vi "Backup File.vi"(7 "Delete Origin File?":bool=TRUE, 8 "error in":errorcluster, 10 "Backup Directory":path, 11 "Original File Path in":path) -> (0 "error out":errorcluster, 3 "Backup File Path out":path)   [LabVIEW 2021, in "EDT File IO.lvlib"]
uses:
  EDT File IO.lvlib
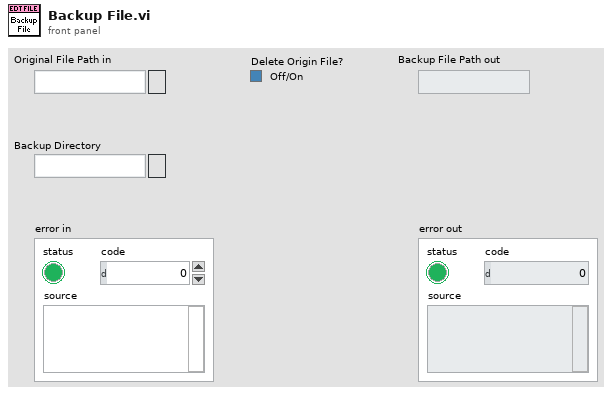
[diagram p1: front panel]
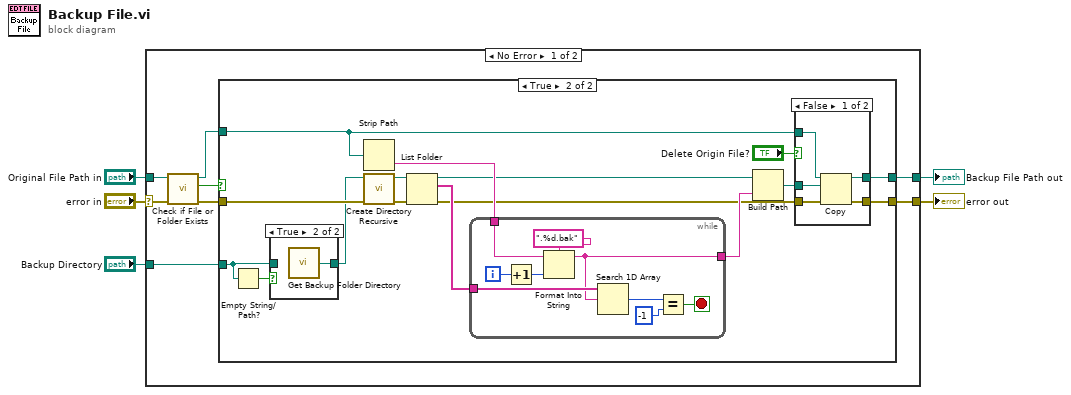
[diagram p0: block diagram]
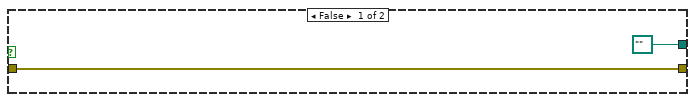
[diagram p2: hidden frame]
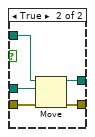
[diagram p3: hidden frame]
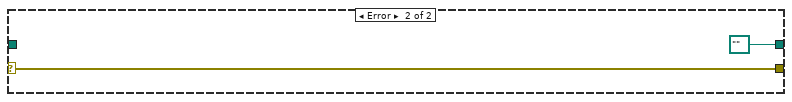
[diagram p5: hidden frame]
diagram:
  n1 = case shown="No Error" "error in" {
    selector: "error in" -> [w9 w54]
    tunnel: [w13 w54] -> w4
    tunnel: [w12 path "" ("File Path in")] -> w3
    tunnel: "Original File Path in" -> [w10 _]
    tunnel: "Backup Directory" -> [w11 _]
    frame No Error {
      n2 = call <vilib>:"Check if File or Folder Exists.vi"("error in (no error)"=w9, "path"=w10) -> ("error out"=w7:errorcluster, "file or folder exists?"=w8:bool, "dup path"=w6:path)  [unwired: 7 in]
      n3 = case shown="True" w8 {
        tunnel: [w15 w31] -> w13
        tunnel: [path "" ("new path") w30] -> w12
        tunnel: w11 -> [_ w24]
        tunnel: w6 -> [_ w23]
        tunnel: w7 -> [w15 w20]
        frame False {
        }
        frame True {
          n4 = Empty String/Path?(string/path=w24) -> (empty?=w25:bool)
          n5 = case shown="True" w25 {
            tunnel: [w42 w43] -> w19
            tunnel: w24 -> [w42 _]
            frame False {
            }
            frame True {
              n6 = call "Get Backup Folder Directory.vi"() -> ("Backup Folder Directory"=w43:path)
            }
          }
          n7 = Strip Path(path=w23) -> (name=w28:string)  [unwired: 1 out]
          n8 = call <vilib>:"Create Directory Recursive.vi"("error in (no error)"=w20, "directory"=w19) -> ("error out"=w17:errorcluster, "directory copy"=w18:path)  [unwired: 3 in, 1 out]
          n9 = List Folder(path=w18, error in=w17) -> (path out=w16:path, filenames=w29:string[], error out=w21:errorcluster)  [unwired: 2 in, 1 out]
          n10 = while {
            tunnel: w29 -> [w52]
            tunnel: w28 -> [w46]
            tunnel: [w44] -> w27
            i -> [w48]
            stop <- w49 stop-if-true
            n11 = Increment(x=w48) -> (x+1=w47:i32)
            n12 = Format Into String(format string=".%d.bak", initial string=w46, w47) -> (resulting string=w44:string)  [unwired: 1 in, 1 out]
            n13 = Search 1D Array(1D array=w52, element=w44) -> (index of element=w51:i32)  [unwired: 1 in]
            n14 = Equal?(x=w51, y=-1) -> (x = y?=w49:bool)
          }
          n15 = Build Path(base path=w16, name or relative path=w27) -> (appended path=w26:path)
          n16 = case shown="False" "Delete Origin File?" {
            tunnel: [w36 w41] -> w31
            tunnel: [w35 w40] -> w30
            tunnel: w26 -> [w34 w39]
            tunnel: w23 -> [w33 w38]
            tunnel: w21 -> [w32 w37]
            frame False {
              n17 = Copy(8:w32, 10:w34, 11:w33) -> (0:w36:errorcluster, 3:w35:path)  [unwired: 2 in, 1 out]
            }
            frame True {
              n18 = Move(source path=w38, error in=w37, 10:w39) -> (error out=w41:errorcluster, 3:w40:path)  [unwired: 2 in, 1 out]
            }
          }
        }
      }
    }
    frame Error {
    }
  }
  "Backup File Path out" <- w3
  "error out" <- w4
